vi "OutSineOffsetGet.vi"(0 "SR865 in":T1, 5 "error in":errorcluster) -> (14 "SR865 out":T1, 16 "Offset":dbl caption="Offset, V", 19 "error out":errorcluster)   [LabVIEW 2018]
uses:
  SR865.ctl
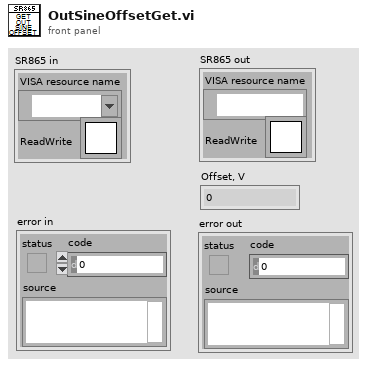
[diagram p1: front panel]
types:
  T1 = typedef "SR865.ctl" = cluster{"VISA resource name":refnum<visa-resource-name>, "ReadWrite":T2}
  T2 = typedef "Semaphore RefNum" = refnum<k1>
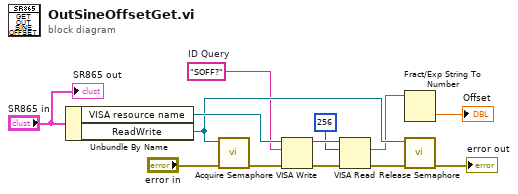
[diagram p0: block diagram]
diagram:
  w1 = "SOFF?"  # ID Query
  n1 = Unbundle By Name("SR865 in") -> ("VISA resource name"=w9:refnum<visa-resource-name>, "ReadWrite"=w4:T2)
  n2 = call <vilib>:"Acquire Semaphore.vi"("error in (no error)"="error in", "semaphore"=w4) -> ("error out"=w8:errorcluster)  [unwired: 3 in, 2 out]
  n3 = VISA Write(VISA resource name=w9, write buffer=w1, error in (no error)=w8) -> (VISA resource name out=w12:refnum<visa-resource-name>, error out=w11:errorcluster)  [unwired: 1 out]
  n4 = VISA Read(VISA resource name=w12, byte count=u32 256, error in (no error)=w11) -> (read buffer=w3:string, error out=w6:errorcluster)  [unwired: 2 out]
  n5 = Fract/Exp String To Number(string=w3) -> (number=→"Offset":dbl)  [unwired: 3 in, 1 out]
  n6 = call <vilib>:"Release Semaphore.vi"("error in (no error)"=w6, "semaphore"=w4) -> ("error out"=→"error out":errorcluster)  [unwired: 4 in, 1 out]
  "SR865 out" <- "SR865 in"
